vi "Logging.vi"(6 "Case":string, 7 "refnum":refnum<file>, 8 "Error In":errorcluster, 10 "Data":string, 11 "Log?":bool) -> (0 "Error Out":errorcluster, 3 "refnum out":refnum<file>)   [LabVIEW 2019]
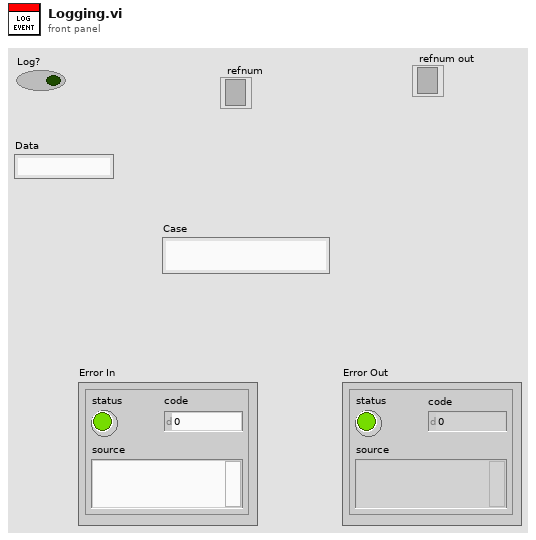
[diagram p1: front panel]
types:
  T1 = enum16{"open", "replace", "create", "open or create", "replace or create", "replace or create with confirmation"}
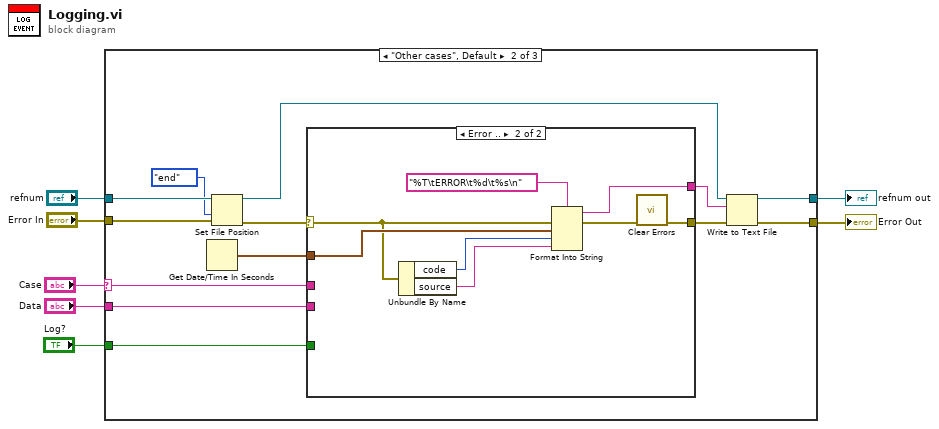
[diagram p0: block diagram]
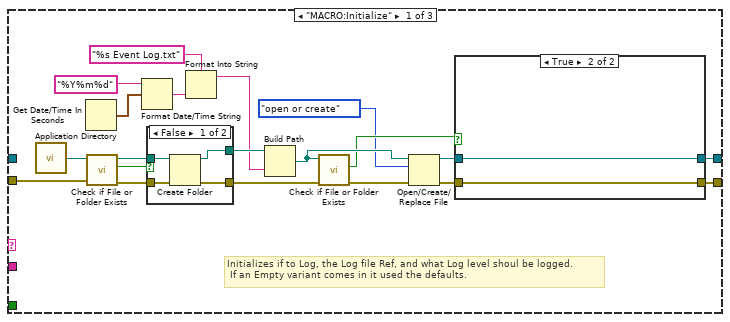
[diagram p2: hidden frame]
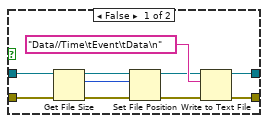
[diagram p4: hidden frame]
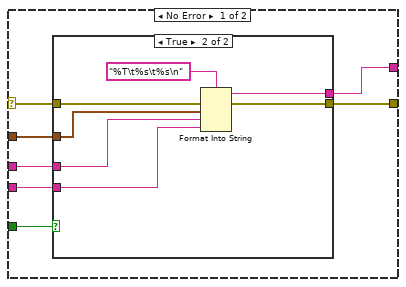
[diagram p5: hidden frame]
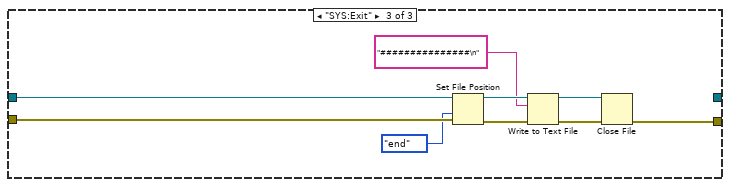
[diagram p7: hidden frame]
diagram:
  n1 = case shown="\"Other cases\", Default" "Case" {
    selector: "Case" -> [_ w55 _]
    tunnel: [w10 w56 w90] -> w7
    tunnel: [w9 w49 _] -> w1
    tunnel: "Log?" -> [_ w48 _]
    tunnel: "Error In" -> [w8 w51 w89]
    tunnel: "Data" -> [_ w50 _]
    tunnel: "refnum" -> [_ w47 w88]
    frame "MACRO:Initialize" {
      # "Initializes if to Log, the Log file Ref, and what Log level shoul be logged.\n If an Empty variant comes in it used the defaults."
      n2 = call <vilib>:"Application Directory.vi"() -> ("Application Directory"=w11:path)
      n3 = Get Date/Time In Seconds() -> (seconds since 1Jan1904=w20:timestamp)
      n4 = call <vilib>:"Check if File or Folder Exists.vi"("error in (no error)"=w8, "path"=w11) -> ("error out"=w22:errorcluster, "file or folder exists?"=w25:bool, "dup path"=w24:path)  [unwired: 7 in]
      n5 = Format Date/Time String(time format string (%c)="%Y%m%d", seconds (now)=w20) -> (date/time string=w19:string)  [unwired: 1 in]
      n6 = case shown="False" w25 {
        tunnel: w24 -> [w31 w33]
        tunnel: [w30 w33] -> w26
        tunnel: w22 -> [w29 w32]
        tunnel: [w28 w32] -> w23
        frame False {
          n7 = Create Folder(path (use dialog)=w31, error in=w29) -> (created path=w30:path, error out=w28:errorcluster)  [unwired: 1 in, 1 out]
        }
        frame True {
        }
      }
      n8 = Format Into String(format string="%s Event Log.txt" ("name or relative path"), w19) -> (resulting string=w18:string)  [unwired: 2 in, 1 out]
      n9 = Build Path(base path=w26, name or relative path=w18) -> (appended path=w17:path)
      n10 = call <vilib>:"Check if File or Folder Exists.vi"("error in (no error)"=w23, "path"=w17) -> ("error out"=w15:errorcluster, "file or folder exists?"=w16:bool)  [unwired: 7 in, 1 out]
      n11 = Open/Create/Replace File(file path (use dialog)=w17, error in=w15, operation (0:open)=T1."open or create") -> (refnum out=w27:refnum<file>, error out=w21:errorcluster)  [unwired: 3 in, 1 out]
      n12 = case shown="True" w16 {
        tunnel: w21 -> [w43 w44]
        tunnel: [w42 w44] -> w10
        tunnel: w27 -> [w38 w45]
        tunnel: [w41 w45] -> w9
        frame False {
          n13 = Get File Size(file=w38, error in=w43) -> (refnum out=w36:refnum<file>, size (in bytes)=w34:i64, 0:w39:errorcluster)
          n14 = Set File Position(offset (in bytes) (0)=w34, refnum=w36, error in=w39) -> (refnum out=w35:refnum<file>, error out=w37:errorcluster)  [unwired: 1 in]
          n15 = Write to Text File(file (use dialog)=w35, text="Data//Time\tEvent\tData\n", error in=w37) -> (refnum out=w41:refnum<file>, error out=w42:errorcluster)  [unwired: 1 in, 1 out]
        }
        frame True {
        }
      }
    }
    frame "Other cases", Default {
      n16 = Get Date/Time In Seconds() -> (seconds since 1Jan1904=w52:timestamp)
      n17 = Set File Position(refnum=w47, from (0:start)=enum16{"start", "end", "current"}."end", error in=w51) -> (refnum out=w53:refnum<file>, error out=w54:errorcluster)  [unwired: 1 in]
      n18 = case shown="Error .." w54 {
        selector: w54 -> [w64 w76]
        tunnel: [w63 w75] -> w58
        tunnel: w52 -> [w65 w77]
        tunnel: [w62 w78] -> w57
        tunnel: w50 -> [w60 _]
        tunnel: w55 -> [w61 _]
        tunnel: w48 -> [w59 _]
        frame No Error {
          n19 = case shown="True" w59 {
            tunnel: w65 -> [_ w73]
            tunnel: w64 -> [w66 w72]
            tunnel: [w66 w71] -> w63
            tunnel: [_ w69] -> w62
            tunnel: w61 -> [_ w68]
            tunnel: w60 -> [_ w67]
            frame False {
            }
            frame True {
              n20 = Format Into String(format string="%T\t%s\t%s\n", error in=w72, w73, w68, w67) -> (resulting string=w69:string, error out=w71:errorcluster)  [unwired: 1 in]
            }
          }
        }
        frame Error {
          n21 = Unbundle By Name(w76) -> ("code"=w81:i32, "source"=w80:string)
          n22 = Format Into String(format string="%T\tERROR\t%d\t%s\n", error in=w76, w77, w81, w80) -> (resulting string=w78:string, error out=w74:errorcluster)  [unwired: 1 in]
          n23 = call <vilib>:"Clear Errors.vi"("error in (no error)"=w74) -> ("error out"=w75:errorcluster)  [unwired: 5 in, 1 out]
        }
      }
      n24 = Write to Text File(file (use dialog)=w53, text=w57, error in=w58) -> (refnum out=w49:refnum<file>, error out=w56:errorcluster)  [unwired: 1 in, 1 out]
    }
    frame "SYS:Exit" {
      n25 = Set File Position(refnum=w88, from (0:start)=enum16{"start", "end", "current"}."end", error in=w89) -> (refnum out=w86:refnum<file>, error out=w85:errorcluster)  [unwired: 1 in]
      n26 = Write to Text File(file (use dialog)=w86, text="###############\n", error in=w85) -> (refnum out=w87:refnum<file>, error out=w83:errorcluster)  [unwired: 1 in, 1 out]
      n27 = Close File(refnum=w87, error in=w83) -> (error out=w90:errorcluster)  [unwired: 1 out]
    }
  }
  "Error Out" <- w7
  "refnum out" <- w1
